vi "Square wave generator.vi"() -> ()   [LabVIEW 2013]
uses:
  Control 2.ctl
  Control 3.ctl
  Control 4.ctl
  Control 5.ctl
  Control 6.ctl
panel:
  in  "Bit 16":T1
  in  "Bit 15":T2
  in  "Bit 14":T3
  in  "Bit 13":T4
  in  "Bit 12":T5
  in  "Bit 11":bool
  in  "Bit 9 - Cell on (inv.)":bool
  in  "Bit 10":bool
  in  "Bit 8":bool
  in  "Bit 7":bool
  in  "Bit 6":bool
  in  "Bit 5":bool
  in  "Bit 4":bool
  in  "Bit 3":bool
  in  "Bit 1":bool
  in  "Bit 2":bool
  in  "Stop":bool
  in  "DAC output (V) 2":dbl(slide) scale=0.0..4.8
  in  "DAC output (V)":dbl(slide) scale=0.0..4.8
  in  "Wait (ms)":u32
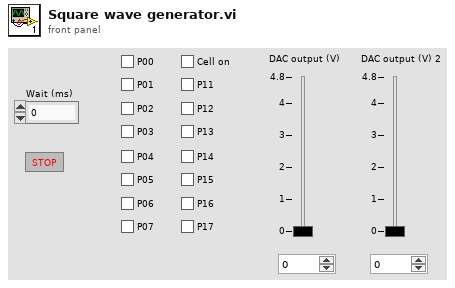
[diagram p1: front panel]
types:
  T1 = typedef "Control 6.ctl" = bool
  T2 = typedef "Control 5.ctl" = bool
  T3 = typedef "Control 4.ctl" = bool
  T4 = typedef "Control 3.ctl" = bool
  T5 = typedef "Control 2.ctl" = bool
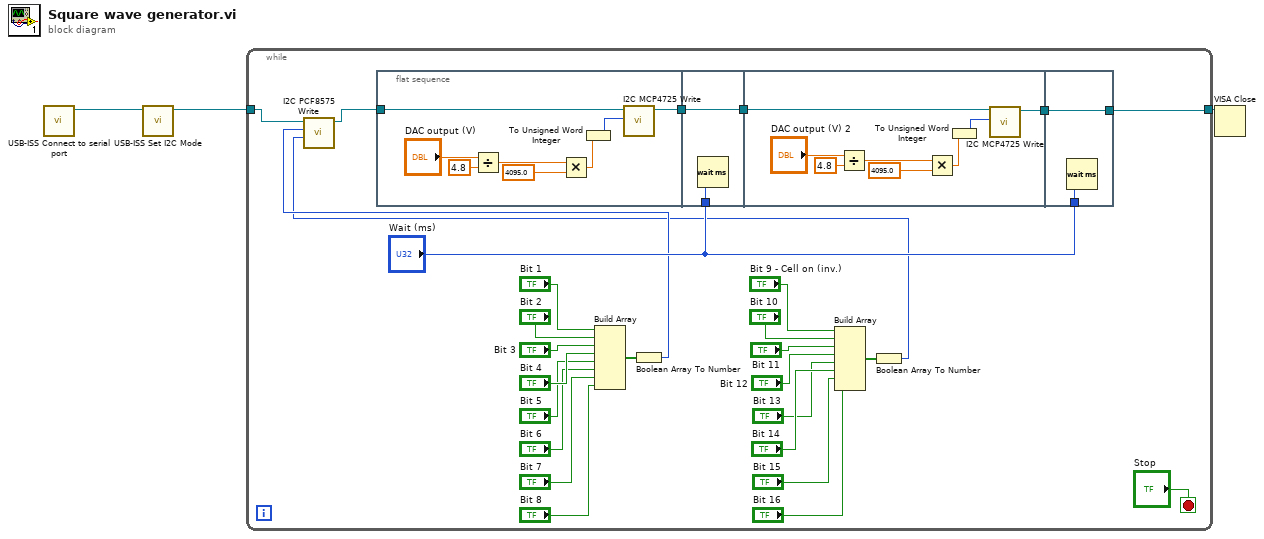
[diagram p0: block diagram]
diagram:
  n1 = call "USB-ISS Connect to serial port.vi"() -> ("VISA Refnum out"=w3:refnum<visa-resource-name>)  [unwired: 10 in, 1 out]
  n2 = call "USB-ISS Set I2C Mode.vi"("VISA Refnum in"=w3) -> ("VISA Refnum out"=w2:refnum<visa-resource-name>)  [unwired: 9 in, 1 out]
  n3 = while {
    tunnel: w2 -> [w7]
    tunnel: [w27] -> w1
    stop <- "Stop" stop-if-true
    n4 = flat-sequence {
      tunnel: w6 -> [w33]
      tunnel: [w32] -> w29
      tunnel: "Wait (ms)" -> [w41]
      tunnel: [w40] -> w30
      tunnel: w29 -> [w40]
      tunnel: w30 -> [w43]
      tunnel: [w42] -> w28
      tunnel: "Wait (ms)" -> [w51]
      tunnel: [w50] -> w27
      tunnel: w28 -> [w50]
      frame #0 {
        n5 = Divide(x="DAC output (V)", y=4.8) -> (x/y=w37:dbl)
        n6 = Multiply(x=w37, y=4095.0) -> (x*y=w35:dbl)
        n7 = To Unsigned Word Integer(number=w35) -> (unsigned 16bit integer=w34:u16)
        n8 = call "I2C MCP4725 Write.vi"("DAC code"=w34, "VISA Refnum in"=w33) -> ("VISA Refnum out"=w32:refnum<visa-resource-name>)  [unwired: 6 in, 1 out]
      }
      frame #1 {
        n9 = Wait (ms)(milliseconds to wait=w41) -> ()  [unwired: 1 out]
      }
      frame #2 {
        n10 = Divide(x="DAC output (V) 2", y=4.8) -> (x/y=w47:dbl)
        n11 = Multiply(x=w47, y=4095.0) -> (x*y=w45:dbl)
        n12 = To Unsigned Word Integer(number=w45) -> (unsigned 16bit integer=w44:u16)
        n13 = call "I2C MCP4725 Write.vi"("DAC code"=w44, "VISA Refnum in"=w43) -> ("VISA Refnum out"=w42:refnum<visa-resource-name>)  [unwired: 6 in, 1 out]
      }
      frame #3 {
        n14 = Wait (ms)(milliseconds to wait=w51) -> ()  [unwired: 1 out]
      }
    }
    n15 = Build Array("Bit 1", "Bit 2", "Bit 3", "Bit 4", "Bit 5", "Bit 6", "Bit 7", "Bit 8") -> (w25:bool[])
    n16 = Boolean Array To Number(Boolean array=w25) -> (number=w5:u8)
    n17 = Build Array("Bit 9 - Cell on (inv.)", "Bit 10", "Bit 11", "Bit 12", "Bit 13", "Bit 14", "Bit 15", "Bit 16") -> (w16:T1[])
    n18 = Boolean Array To Number(Boolean array=w16) -> (number=w4:u8)
    n19 = call "I2C PCF8575 Write.vi"("Byte 2"=w4, "Byte 1"=w5, "VISA Refnum in"=w7) -> ("VISA Refnum out"=w6:refnum<visa-resource-name>)  [unwired: 7 in, 1 out]
  }
  n20 = VISA Close(VISA resource name=w1) -> ()  [unwired: 1 in, 1 out]
